vi "Configure Channels.vi"(8 "error in":errorcluster, 11 "DO DAQmx Fixed Freq PWM CFG in":refnum<class "DO DAQmx Fixed Freq PWM CFG.lvclass">) -> (0 "error out":errorcluster, 3 "DO DAQmx Fixed Freq PWM CFG out":refnum<class "DO DAQmx Fixed Freq PWM CFG.lvclass">)   [LabVIEW 2023, in "DO DAQmx Fixed Freq PWM CFG.lvclass"]
uses:
  DO DAQmx Fixed Freq PWM CFG.lvclass
  Configuration/Configuration JSON/Configuration JSON Base/CFG JSON.lvclass/CFG JSON.ctl
  DO DAQmx Fixed Freq PWM CFG.lvclass/DO DAQmx Fixed Freq PWM CFG.ctl
  DAQmx/DAQmx Base CFG/DAQmx Base CFG.lvclass/DAQmx Base CFG.ctl
  <vilib>/Utility/miscctls.llb/LVMapReplaceAction.ctl
  6411cd84-0cc3-40a4-b609-a223cd4ed0c4.vi
  <vilib>/JDP Science/JSONtext/Find Item.vi
  <vilib>/JDP Science/JSONtext/Next JSON Value.vi
  <vilib>/JDP Science/JSONtext/String Subset.vi
  <vilib>/JDP Science/JSONtext/Parsing/Advance past next JSON Value (inlined COPY).vi
  <vilib>/JDP Science/JSONtext/Parsing/Advance past whitespace.vi
  <vilib>/JDP Science/JSONtext/Parsing/Advance past String.vi
  <vilib>/JDP Science/JSONtext/Parsing/Advance past Number.vi
  <vilib>/JDP Science/JSONtext/Parsing/Advance past Line Ending.vi
  <vilib>/JDP Science/JSONtext/Parsing/Parse Full Path or Item Name.vi
  <vilib>/JDP Science/JSONtext/Parsing/Advance past Array.vi
  <vilib>/JDP Science/JSONtext/Parsing/Advance past Object.vi
  <vilib>/JDP Science/JSONtext/support/Error Cluster From Code.vi
  <vilib>/JDP Science/JSONtext/Offset/Find Item Locations by Path.vi
  <vilib>/JDP Science/JSONtext/JSON text to Variant.vi
  <vilib>/Utility/error.llb/Error Cluster From Error Code.vi
  <vilib>/DAQmx/create/channels.llb/DAQmx Create Channel (DO-Digital Output).vi
  <vilib>/JDP Science/JSONtext/LVClass Serializer/JSONtext LVClass Serializer.lvclass
  <vilib>/ErrorRing/Error Ring.xnode
  DAQmx/DAQmx Base CFG/DAQmx Base CFG.lvclass
  Configuration/Configuration JSON/Configuration JSON Base/CFG JSON.lvclass
  <resource>/objmgr/daqmx.rc
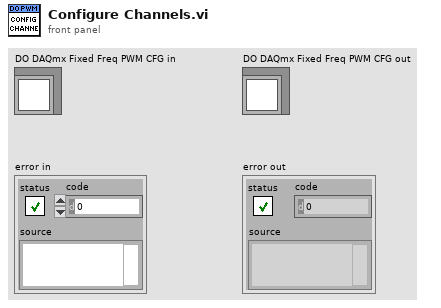
[diagram p1: front panel]
types:
  T1 = cluster{"Name":string, "Enabled":bool, "Frequency":dbl, "Duty Cycle":dbl, "Invert Lines":bool}[]
  T2 = typedef "LVMapReplaceAction.ctl" = enum32{"Modify Entry only if found", "Add or Modify Entry", "Delete Entry"}
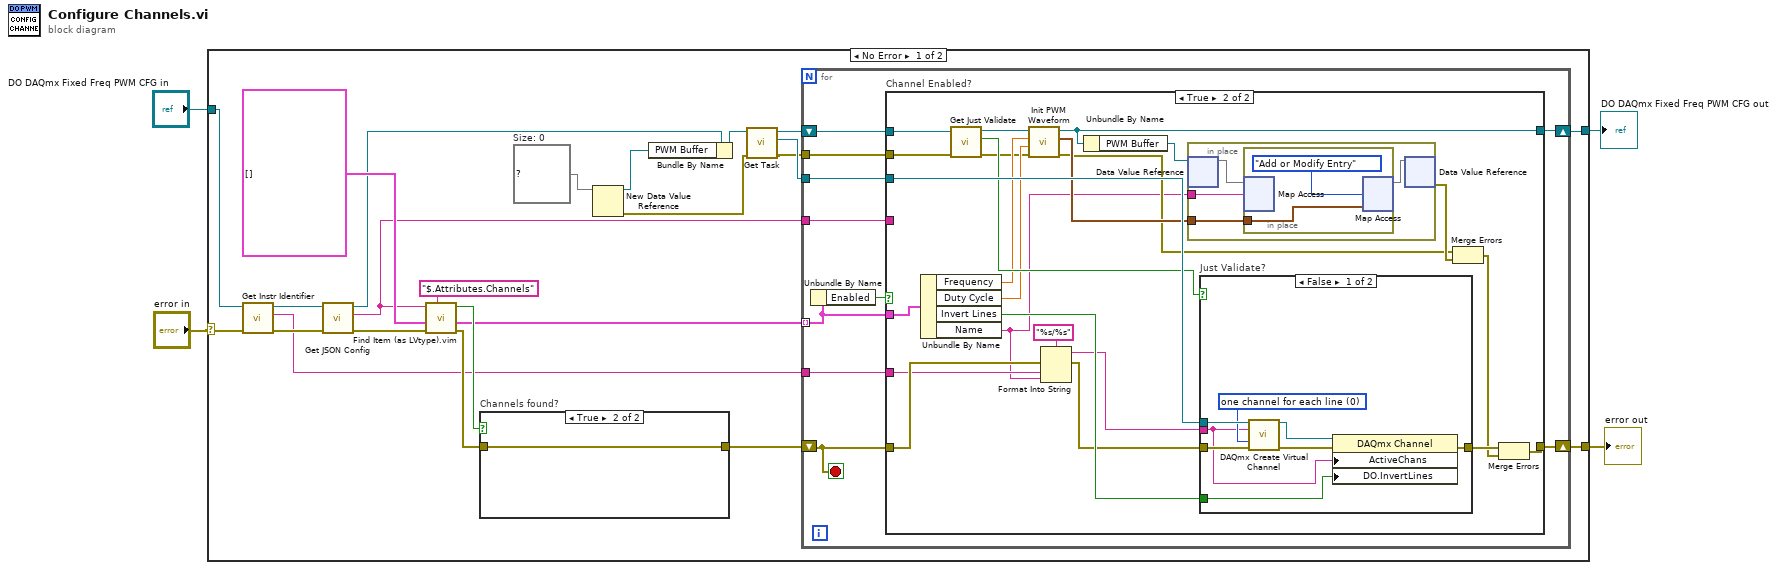
[diagram p0: block diagram]
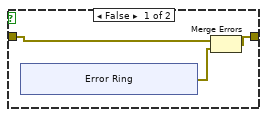
[diagram p2: hidden frame]
diagram:
  n1 = case shown="No Error" "error in" {
    selector: "error in" -> [w18 w88]
    tunnel: "DO DAQmx Fixed Freq PWM CFG in" -> [w13 w89]
    tunnel: [w19 w88] -> w2
    tunnel: [w12 w89] -> w1
    frame No Error {
      w8 = map{string, digitalwaveform} {}  # Size: 0
      n2 = call-dynamic "Get Instr Identifier.vi"("error in (no error)"=w18, "Configuration Base in"=w13) -> ("error out"=w22:errorcluster, "Instr Ident"=w20:string, "Configuration Base out"=w21:refnum<class "DO DAQmx Fixed Freq PWM CFG.lvclass">)  [unwired: 7 in]
      n3 = call "Get JSON Config.vi"("error in (no error)"=w22, "CFG Base in"=w21) -> ("error out"=w26:errorcluster, "<JSON>Config>"=w17:string, "CFG Base out"=w15:refnum<class "DO DAQmx Fixed Freq PWM CFG.lvclass">)  [unwired: 7 in]
      n4 = call "Find Item (as LVtype).vim"("$Path or Item Name"="$.Attributes.Channels", "error in (no error)"=w26, "Data Type and Default Value"=T1 [], "JSON"=w17) -> ("error out"=w24:errorcluster, "Data"=w14:T1, "Found"=w25:bool)  [unwired: 4 in, 1 out]
      n5 = case "Channels found?" shown="True" w25 {
        tunnel: w24 -> [w30 w36]
        tunnel: [w28 w36] -> w9
        frame False {
          n6 = xnode "Error Ring"() -> ("error out"=w29:errorcluster)
          n7 = Merge Errors(w30, w29) -> (w28:errorcluster)
        }
        frame True {
        }
      }
      n8 = New Data Value Reference(data value=w8) -> (data value reference=w5:refnum<data-value>, error out=w7:errorcluster)  [unwired: 1 in]
      n9 = Bundle By Name(cluster=w15, "PWM Buffer"=w5) -> (w6:refnum<class "DO DAQmx Fixed Freq PWM CFG.lvclass">)
      n10 = call "Get Task.vi"("error in"=w7, "DAQmx Base CFG in"=w6) -> ("error out"=w10:errorcluster, "Task"=w16:refnum<k21>, "DAQmx Base CFG out"=w11:refnum<class "DO DAQmx Fixed Freq PWM CFG.lvclass">)  [unwired: 7 in]
      n11 = for {
        tunnel: w14 -> [w43] mode=indexing
        shift-right: [w46] -> w19
        shift-left: w9 -> [w45]
        tunnel: w20 -> [w44]
        tunnel: w17 -> [w41]
        tunnel: w16 -> [w40]
        shift-right: [w39] -> w12
        shift-left: w11 -> [w38]
        tunnel: w10 -> [w37]
        stop <- w45 stop-if-true
        n12 = Unbundle By Name(w43) -> ("Enabled"=w42:bool)
        n13 = case "Channel Enabled?" shown="True" w42 {
          tunnel: [w48 w68] -> w46
          tunnel: w45 -> [w48 w57]
          tunnel: w44 -> [_ w55]
          tunnel: w43 -> [_ w72]
          tunnel: [w47 w50] -> w39
          tunnel: w41 -> [_ _]
          tunnel: w40 -> [_ w65]
          tunnel: w38 -> [w47 w64]
          tunnel: w37 -> [_ w56]
          frame False {
          }
          frame True {
            n14 = Unbundle By Name(w72) -> ("Frequency"=w60:dbl, "Duty Cycle"=w59:dbl, "Invert Lines"=w70:bool, "Name"=w49:string)
            n15 = call "Get Just Validate.vi"("error in (no error)"=w56, "CFG JSON Base in"=w64) -> ("error out"=w52:errorcluster, "Just Validate"=w62:bool, "CFG JSON Base out"=w63:refnum<class "DO DAQmx Fixed Freq PWM CFG.lvclass">)  [unwired: 7 in]
            n16 = call-dynamic "Init PWM Waveform.vi"("error in"=w52, "Duty Cycle"=w59, "Frequency"=w60, "DO DAQmx Fixed Freq PWM CFG in"=w63) -> ("error out"=w51:errorcluster, "PWM Waveform"=w61:digitalwaveform, "DO DAQmx Fixed Freq PWM CFG out"=w50:refnum<class "DO DAQmx Fixed Freq PWM CFG.lvclass">)  [unwired: 5 in]
            n17 = Format Into String(format string="%s/%s", error in=w57, w55, w49) -> (resulting string=w53:string, error out=w54:errorcluster)  [unwired: 1 in]
            n18 = Unbundle By Name(w50) -> ("PWM Buffer"=w69:refnum<data-value>)
            n19 = in-place {
              in-place-border: w49 -> [w75]
              in-place-border: w61 -> [w74]
              n20 = in-place-dvr #1(w69) -> (w76:map{string, digitalwaveform})  [unwired: 1 out]
              n21 = in-place {
                in-place-border: w74 -> [w77]
                n22 = in-place-map #2(w76, w75) -> ()  [unwired: 1 in, 2 out]
                n23 = in-place-map #2(w77, LVMapReplaceAction."Add or Modify Entry" ("action")) -> (w73:map{string, digitalwaveform})  [unwired: 2 out]
              }
              n24 = in-place-dvr #1(w73) -> (w67:errorcluster)  [unwired: 1 out]
            }
            n25 = case "Just Validate?" shown="False" w62 {
              tunnel: w54 -> [w86 w87]
              tunnel: w53 -> [w79 _]
              tunnel: w65 -> [w85 _]
              tunnel: [w83 w87] -> w71
              tunnel: w70 -> [w80 _]
              frame False {
                w81 = 0 items=["one channel for each line", "one channel for all lines"] ("line grouping 2")
                n26 = call-poly <vilib>:"DAQmx Create Virtual Channel.vi"("task in"=w85, "lines"=w79, "line grouping"=w81, "error in"=w86) -> ("task out"=w82:refnum<k21>, "error out"=w84:errorcluster)  [unwired: 10 in]
                n27 = property class="DAQmx Channel"(reference=w82, error in=w84, "ActiveChans"=w79, "DO.InvertLines"=w80) -> (error out=w83:errorcluster)  [unwired: 1 out]
              }
              frame True {
              }
            }
            n28 = Merge Errors(w51, w67) -> (w66:errorcluster)
            n29 = Merge Errors(w71, w66) -> (w68:errorcluster)
          }
        }
      }
    }
    frame Error {
    }
  }
  "error out" <- w2
  "DO DAQmx Fixed Freq PWM CFG out" <- w1
